vi "Create Report CSV.vi"(8 "error in (no error)":errorcluster, 10 "Fixture Name":string, 11 "Report Info":T1={"Serial Number"="PAS123456", "Test Results"={"Vacuum Test"=[{"Functional Pressure"=1.0, "Leak Pressure"=2.0, "Func Pass?"=TRUE, "Leak Pass?"=TRUE, "Step Start"=timestamp(3537898015.259423 s since 1904-01-01), "Step End"=timestamp(0 s since 1904-01-01)}, {"Functional Pressure"=10.0, "Leak Pressure"=5.0, "Func Pass?"=FALSE, "Leak Pass?"=FALSE, "Step Start"=timestamp(3537898225.81034 s since 1904-01-01), "Step End"=timestamp(0 s since 1904-01-01)}], "Helium Test"=[{"Functional Pressure"=0.0, "Leak Pressure"=2.0, "Func Pass?"=FALSE, "Leak Pass?"=FALSE, "Step Start"=timestamp(3537898026.346761 s since 1904-01-01), "Step End"=timestamp(0 s since 1904-01-01)}, {"Functional Pressure"=0.0, "Leak Pressure"=55.0, "Func Pass?"=FALSE, "Leak Pass?"=TRUE, "Step Start"=timestamp(3537898239.0582047 s since 1904-01-01), "Step End"=timestamp(0 s since 1904-01-01)}], "Aborted?"=FALSE, "Reason"="", "Abort Time"=timestamp(0 s since 1904-01-01), "Test Start"=timestamp(0 s since 1904-01-01), "Test End"=timestamp(0 s since 1904-01-01)}, "Test Configuration"={"Vacuum Test"={"Vacuum Timings"=[], "Vacuum Thresholds"=[{"Func Max Pressure"=1.0, "Func Min Pressure"=0.0, "Leak Max Pressure"=2.0, "Leak Min Pressure"=0.0}, {"Func Max Pressure"=1.0, "Func Min Pressure"=0.0, "Leak Max Pressure"=2.0, "Leak Min Pressure"=0.0}], "Leak Reasons"=["GV_1 Failure", "GV_2 Failure"], "Func Reasons"=["GV2_CB Failure", "GV3_CB Failure"], "FuncSpecEqual"=["FuncSpec1.01", "FuncSpec1.02"], "LeakSpecEqual"=["FuncSpec1.02", "FuncSpec1.03"]}, "Helium Test"={"Helium Timings"=[], "Helium Thresholds"=[{"Func Max Pressure"=0.0, "Func Min Pressure"=0.0, "Leak Max Pressure"=23.0, "Leak Min Pressure"=0.0}, {"Func Max Pressure"=0.0, "Func Min Pressure"=0.0, "Leak Max Pressure"=10.0, "Leak Min Pressure"=0.0}], "Failure Reasons"=["Pressure Regulator Failed", "Leak in Fixture at CAL port"], "LeakSpecEqual"=["LeakSpec 1.02", "LeakSpec 1.03"]}, "Functional Test"={"Mic Test ON ADC Max"=0.0, "Mic Test ON ADC Min"=0.0, "Mic Test OFF ADC Max"=0.0, "Mic Test OFF ADC Min"=0.0, "Mic Test IC ADC Max"=0.0, "Mic Test IC ADC Min"=0.0, "IR Emitter ON ADC Max"=0.0, "IR Emitter ON ADC Min"=0.0, "IR Emitter OFF ADC Max"=0.0, "IR Emitter OFF ADC Min"=0.0}}, "Operator"="hvu", "Config Filepath"=path "C:/PAS Circulation Tester/Configuration/testConfig.xml"}) -> (0 "error out":errorcluster)   [LabVIEW 2015]
uses:
  Controls/Report Config.ctl
  Tests/Controls/Test Results.ctl
  Tests/Controls/Step Result.ctl
  Tests/Controls/Test Configuration.ctl
  Tests/Controls/Vacuum Test.ctl
  Tests/Controls/Test Timing.ctl
  Tests/Controls/Vaccum Thresholds.ctl
  Tests/Controls/Helium Test.ctl
  Tests/Controls/Helium Thresholds.ctl
  Tests/Controls/Functional Test.ctl
  <userlib>/_OpenG.lib/file/file.llb/Strip Path Extension - Path__ogtk.vi
panel:
  in  "Columns":string[](array[string])=["SerialNumber", "TestName", "TimeStamp", "SpecName", "ResultValue", "SpecMin", "SpecMax", "ResultText", "SpecEqual", "SpecUnit", "PassFail", "UserName"]
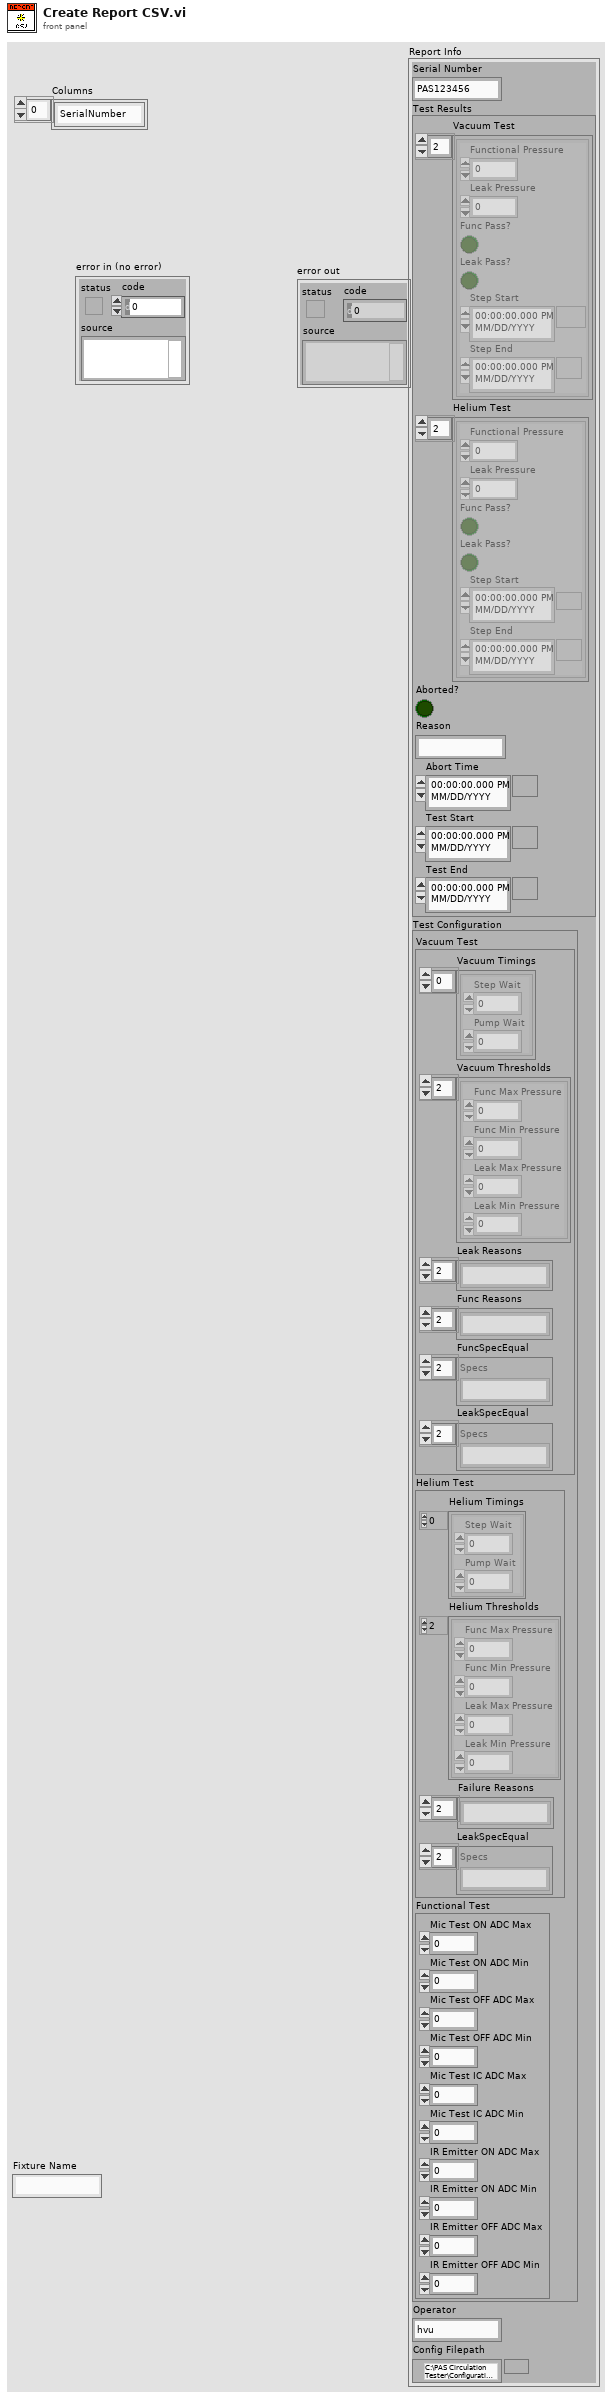
[diagram p1: front panel]
types:
  T1 = typedef "Report Config.ctl" = cluster{"Serial Number":string, "Test Results":T2, "Test Configuration":T4, "Operator":string, "Config Filepath":path}
  T2 = typedef "Test Results.ctl" = cluster{"Vacuum Test":T3[], "Helium Test":T3[], "Aborted?":bool, "Reason":string, "Abort Time":timestamp, "Test Start":timestamp, "Test End":timestamp}
  T3 = typedef "Step Result.ctl" = cluster{"Functional Pressure":dbl, "Leak Pressure":dbl, "Func Pass?":bool, "Leak Pass?":bool, "Step Start":timestamp, "Step End":timestamp}
  T4 = typedef "Test Configuration.ctl" = cluster{"Vacuum Test":T5, "Helium Test":T8, "Functional Test":T10}
  T5 = typedef "Vacuum Test.ctl" = cluster{"Vacuum Timings":T6[], "Vacuum Thresholds":T7[], "Leak Reasons":string[], "Func Reasons":string[], "FuncSpecEqual":string[], "LeakSpecEqual":string[]}
  T6 = typedef "Test Timing.ctl" = cluster{"Step Wait":dbl, "Pump Wait":dbl}
  T7 = typedef "Vaccum Thresholds.ctl" = cluster{"Func Max Pressure":dbl, "Func Min Pressure":dbl, "Leak Max Pressure":dbl, "Leak Min Pressure":dbl}
  T8 = typedef "Helium Test.ctl" = cluster{"Helium Timings":T6[], "Helium Thresholds":T9[], "Failure Reasons":string[], "LeakSpecEqual":string[]}
  T9 = typedef "Helium Thresholds.ctl" = cluster{"Func Max Pressure":dbl, "Func Min Pressure":dbl, "Leak Max Pressure":dbl, "Leak Min Pressure":dbl}
  T10 = typedef "Functional Test.ctl" = cluster{"Mic Test ON ADC Max":dbl, "Mic Test ON ADC Min":dbl, "Mic Test OFF ADC Max":dbl, "Mic Test OFF ADC Min":dbl, "Mic Test IC ADC Max":dbl, "Mic Test IC ADC Min":dbl, "IR Emitter ON ADC Max":dbl, "IR Emitter ON ADC Min":dbl, "IR Emitter OFF ADC Max":dbl, "IR Emitter OFF ADC Min":dbl}
  T11 = enum16{"open", "replace", "create", "open or create", "replace or create", "replace or create with confirmation"}
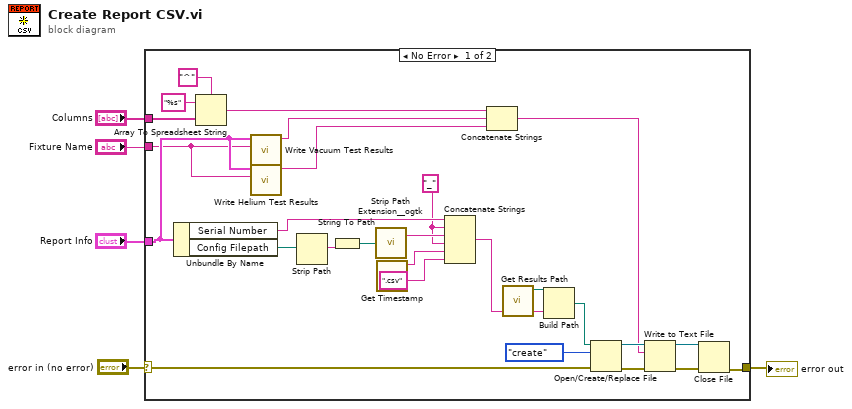
[diagram p0: block diagram]
diagram:
  n1 = case shown="No Error" "error in (no error)" {
    selector: "error in (no error)" -> [w32 w33]
    tunnel: [w21 w33] -> w5
    tunnel: "Report Info" -> [w11 _]
    tunnel: "Columns" -> [w28 _]
    tunnel: "Fixture Name" -> [w6 _]
    frame No Error {
      w7 = "_" ("string")
      n2 = Unbundle By Name(w11) -> ("Serial Number"=w8:string, "Config Filepath"=w18:path)
      n3 = Array To Spreadsheet String(delimiter (Tab)="^", array=w28, 3:"%s" ("format string")) -> (spreadsheet string=w19:string)
      n4 = call "Write Vacuum Test Results.vi"("Fixture Name"=w6, "Report Info"=w11) -> ("String"=w12:string)  [unwired: 8 in, 1 out]
      n5 = call "Write Helium Test Results.vi"("Fixture Name"=w6, "Report Info"=w11) -> ("String"=w10:string)  [unwired: 8 in, 1 out]
      n6 = Strip Path(path=w18) -> (name=w17:string)  [unwired: 1 out]
      n7 = String To Path(string=w17) -> (path=w16:path)
      n8 = call-poly <userlib>:"Strip Path Extension__ogtk.vi"("path"=w16) -> ("root"=w15:string)  [unwired: 1 out]
      n9 = call "Get Timestamp.vi"() -> ("result string"=w14:string)  [unwired: 11 in]
      n10 = Concatenate Strings(w8, w7, w15, w7, w14, ".csv" ("string")) -> (w9:string)
      n11 = Concatenate Strings(w19, w12, w10) -> (w20:string)
      n12 = call "Get Results Path.vi"() -> ("Result Path"=w31:path)  [unwired: 11 in]
      n13 = Build Path(base path=w31, name or relative path=w9) -> (appended path=w30:path)
      n14 = Open/Create/Replace File(file path (use dialog)=w30, error in=w32, operation (0:open)=T11."create") -> (refnum out=w24:refnum<file>, error out=w25:errorcluster)  [unwired: 3 in, 1 out]
      n15 = Write to Text File(file (use dialog)=w24, text=w20, error in=w25) -> (refnum out=w22:refnum<file>, error out=w23:errorcluster)  [unwired: 1 in, 1 out]
      n16 = Close File(refnum=w22, error in=w23) -> (error out=w21:errorcluster)  [unwired: 1 out]
    }
    frame Error {
    }
  }
  "error out" <- w5
